vi "endEventToStringArray.vi"(8 "error in (no error)":errorcluster, 11 "RfRamp in":refnum<class "RfRamp.lvclass">) -> (0 "error out":errorcluster, 2 "eventStringArray":string[](array[string]), 3 "RfRamp out":refnum<class "RfRamp.lvclass">)   [LabVIEW 2009, in "Tools.lvlib" / "Scripting.lvlib" / "RfRamp.lvclass"]
uses:
  RfRamp.lvclass
  RfRamp.lvclass/RfRamp.ctl
  ScriptEvent.lvclass
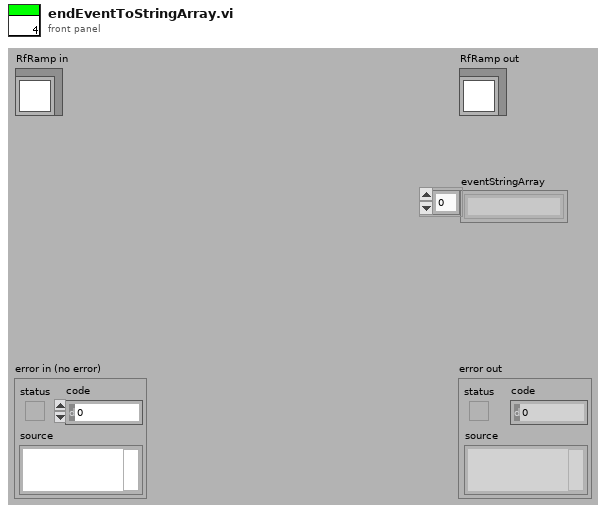
[diagram p1: front panel]
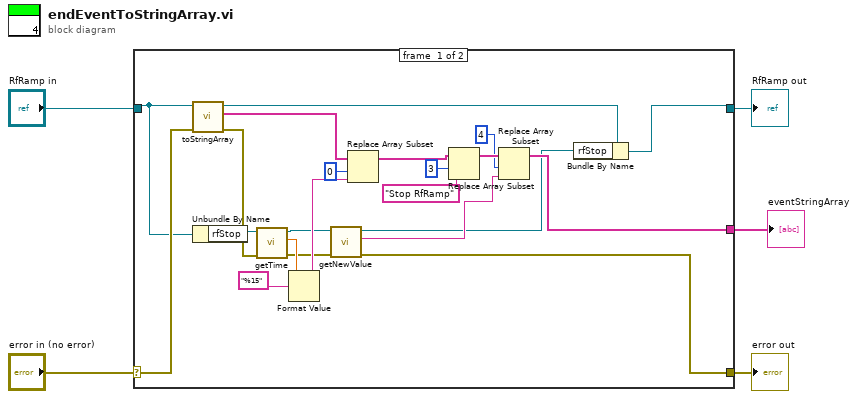
[diagram p0: block diagram]
diagram:
  n1 = case shown="No Error" "error in (no error)" {
    selector: "error in (no error)" -> [w27 w29]
    tunnel: [w11 w29] -> w4
    tunnel: [w14 w28] -> w2
    tunnel: "RfRamp in" -> [w21 w28]
    tunnel: [w7 _] -> w1
    frame #0 {
      n2 = call-dynamic "toStringArray.vi"("error in (no error)"=w27, "RfRamp in"=w21) -> ("error out"=w16:errorcluster, "eventStringArray"=w23:string[], "RfRamp out"=w15:refnum<class "RfRamp.lvclass">)  [unwired: 7 in]
      n3 = Unbundle By Name(w21) -> ("rfStop"=w20:refnum<class "rf.lvclass">)
      n4 = call "getTime.vi"("error in (no error)"=w16, "ScriptEvent.lvclass in"=w20) -> ("error out"=w12:errorcluster, "time"=w19:dbl, "ScriptEvent.lvclass out"=w13:refnum<class "rf.lvclass">)  [unwired: 7 in]
      n5 = Format Value(format string="%15", value (0)=w19) -> (output string=w17:string)  [unwired: 1 in]
      n6 = call "getNewValue.vi"("error in (no error)"=w12, "ScriptEvent.lvclass in"=w13) -> ("error out"=w11:errorcluster, "newValue"=w8:string, "ScriptEvent.lvclass out"=w6:refnum<class "rf.lvclass">)  [unwired: 7 in]
      n7 = Replace Array Subset(array=w23, new element=w17, index=0) -> (w22:string[])
      n8 = Replace Array Subset(array=w22, new element="Stop RfRamp", index=3) -> (w10:string[])
      n9 = Replace Array Subset(array=w10, new element=w8, index=4) -> (w7:string[])
      n10 = Bundle By Name(cluster=w15, "rfStop"=w6) -> (w14:refnum<class "RfRamp.lvclass">)
    }
    frame #1 {
    }
  }
  "error out" <- w4
  "RfRamp out" <- w2
  "eventStringArray" <- w1
